vi "2D String Array_CheckIfEmpty.vi"(2 "2D String Array In":string[][](array[string])) -> (6 "empty?":bool)   [LabVIEW 2020]
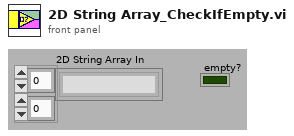
[diagram p1: front panel]
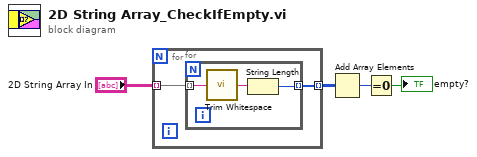
[diagram p0: block diagram]
diagram:
  n1 = for {
    tunnel: "2D String Array In" -> [w6] mode=indexing
    tunnel: [w5] -> w3 mode=indexing
    n2 = for {
      tunnel: w6 -> [w9] mode=indexing
      tunnel: [w7] -> w5 mode=indexing
      n3 = call <vilib>:"Trim Whitespace.vi"("string"=w9) -> ("trimmed string"=w8:string)  [unwired: 1 in]
      n4 = String Length(string=w8) -> (length=w7:i32)
    }
  }
  n5 = Add Array Elements(numeric array=w3) -> (sum=w2:i32)
  n6 = Equal To 0?(x=w2) -> (x = 0?=→"empty?":bool)
